vi "Write mode.vi"(8 "error in (no error)":errorcluster, 10 "wsMode":T1, 11 "WSMode.lvclass in":refnum<class "WSMode.lvclass">) -> (0 "error out":errorcluster, 3 "WSMode.lvclass out":refnum<class "WSMode.lvclass">)   [LabVIEW 2022 SP3, in "TCSDataDefinitions.lvlib" / "TCSWeatherServerCommand.lvlib" / "WSMode.lvclass"]
uses:
  WSMode.lvclass
  Enumerations/wsMode.ctl
  WSMode.lvclass/WSMode.ctl
  TCSWeatherServerCommand.lvlib
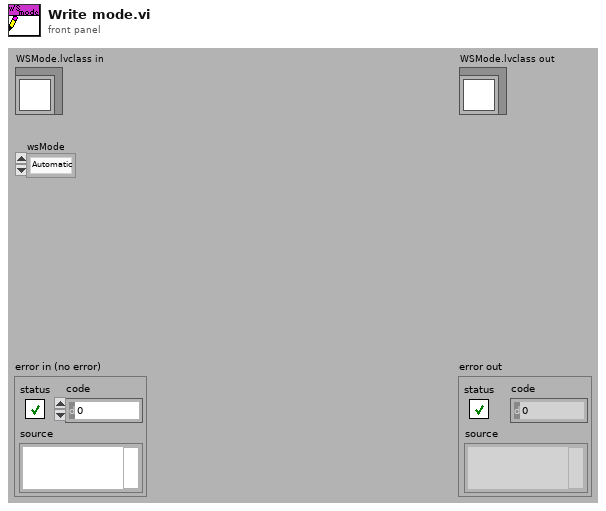
[diagram p1: front panel]
types:
  T1 = typedef "TCSDataDefinitions.lvlib/TCSWeatherServerCommand.lvlib/wsMode.ctl" = enum16{"Automatic", "Manual"}
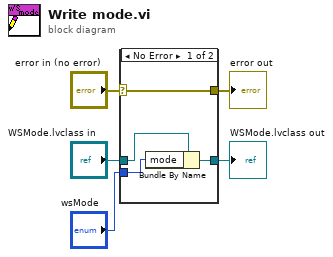
[diagram p0: block diagram]
diagram:
  n1 = case shown="No Error" "error in (no error)" {
    selector: "error in (no error)" -> [w9 w10]
    tunnel: [w9 w10] -> w4
    tunnel: [w7 w11] -> w2
    tunnel: "WSMode.lvclass in" -> [w8 w11]
    tunnel: "wsMode" -> [w6 _]
    frame No Error {
      n2 = Bundle By Name(cluster=w8, "mode"=w6) -> (w7:refnum<class "WSMode.lvclass">)
    }
    frame Error {
    }
  }
  "error out" <- w4
  "WSMode.lvclass out" <- w2
